vi "Control Panel Controller.vi"(8 "error in (no error)":errorcluster, 11 "Control Panel in":refnum<class "Control Panel.lvclass">) -> (0 "error out":errorcluster, 2 "Solenoid":bool, 3 "Control Panel out":refnum<class "Control Panel.lvclass">)   [LabVIEW 2019, in "Control Panel.lvlib" / "Control Panel.lvclass"]
uses:
  Control Panel.lvclass
  Controls/Control Panel State.ctl
panel:
  in  "Rotation":bool
  in  "Position":bool
  in  "Manual":dbl
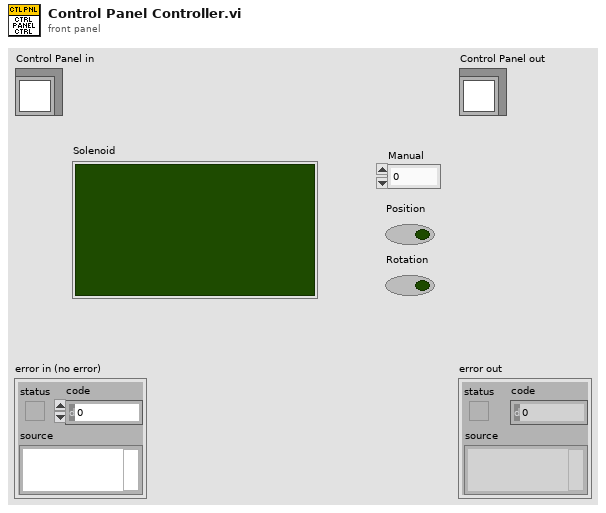
[diagram p1: front panel]
types:
  T1 = typedef "Control Panel State.ctl" = enum16{"Manual Control", "Position Control", "Rotation Control", "Retracted", "Deployed"}
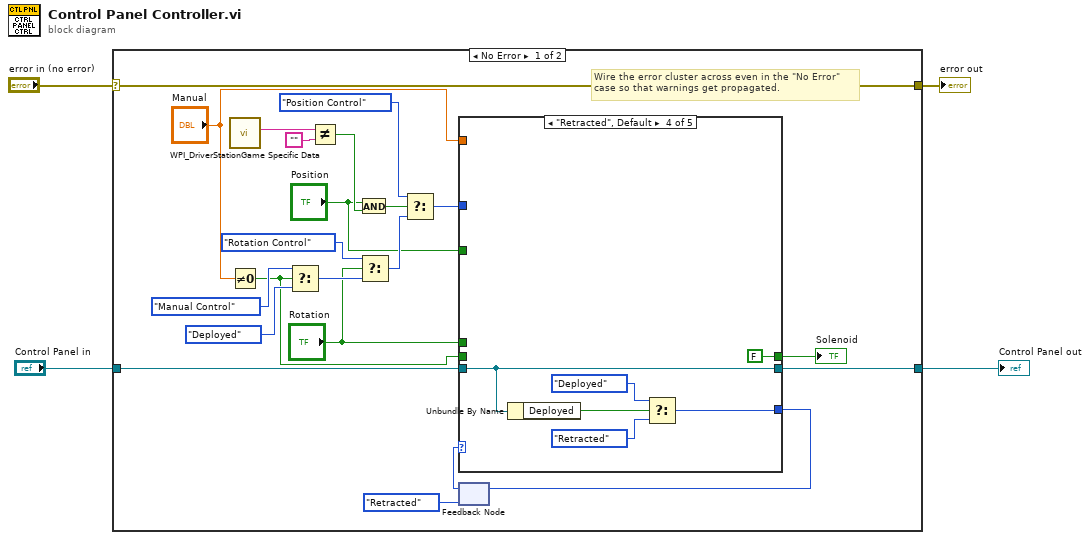
[diagram p0: block diagram]
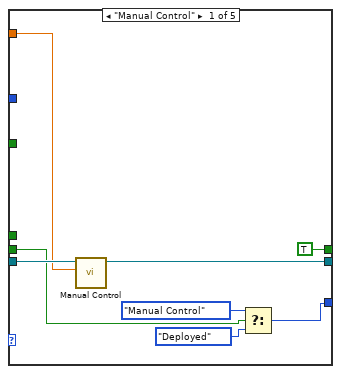
[diagram p2: hidden frame]
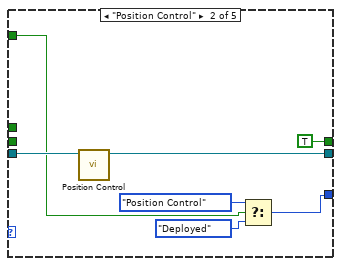
[diagram p3: hidden frame]
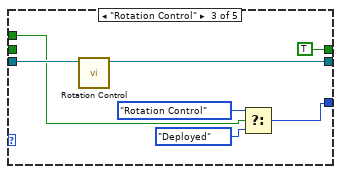
[diagram p4: hidden frame]
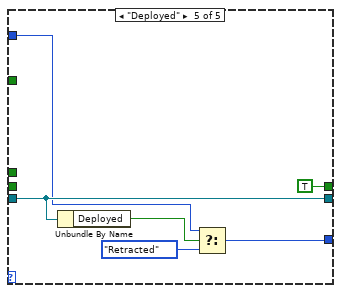
[diagram p5: hidden frame]
diagram:
  n1 = case shown="No Error" "error in (no error)" {
    selector: "error in (no error)" -> [w26 w62]
    tunnel: [w26 w62] -> w3
    tunnel: [w22 w61] -> w1
    tunnel: "Control Panel in" -> [w23 w61]
    frame No Error {
      # "Wire the error cluster across even in the \"No Error\"\ncase so that warnings get propagated."
      n2 = call <vilib>:"WPI_DriverStationGame Specific Data.vi"() -> ("Game Specific Data"=w13:string)  [unwired: 11 in]
      n3 = Not Equal To 0?(x="Manual") -> (x != 0?=w6:bool)
      n4 = Select(t=Control_Panel_State."Manual Control", s=w6, f=Control_Panel_State."Deployed") -> (s? t:f=w18:T1)
      n5 = Not Equal?(x=w13, y="") -> (x != y?=w11:bool)
      n6 = And(x="Position", y=w11) -> (x .and. y?=w5:bool)
      n7 = Select(t=Control_Panel_State."Rotation Control", s="Rotation", f=w18) -> (s? t:f=w19:T1)
      n8 = Select(t=Control_Panel_State."Position Control", s=w5, f=w19) -> (s? t:f=w10:T1)
      n9 = feedback #1(Control_Panel_State."Retracted") -> (w24:T1)
      n10 = case shown="\"Retracted\", Default" w24 {
        tunnel: w23 -> [w34 w41 w48 w51 w59]
        tunnel: [w27 w37 w42 w51 w59] -> w22
        tunnel: [w29 w38 w44 w54 w55] -> w20
        tunnel: [TRUE ("Deployed") TRUE ("Deployed") TRUE ("Deployed") FALSE ("Deployed") TRUE ("Deployed")] -> w21
        tunnel: w10 -> [_ _ _ _ w56]
        tunnel: "Rotation" -> [_ _ w47 _ _]
        tunnel: "Position" -> [_ w36 _ _ _]
        tunnel: "Manual" -> [w33 _ _ _ _]
        tunnel: w6 -> [w32 _ _ _ _]
        frame "Manual Control" {
          n11 = call-dynamic "Manual Control.vi"("Output"=w33, "Control Panel in"=w34) -> ("Control Panel out"=w27:refnum<class "Control Panel.lvclass">)  [unwired: 8 in, 1 out]
          n12 = Select(t=Control_Panel_State."Manual Control", s=w32, f=Control_Panel_State."Deployed") -> (s? t:f=w29:T1)
        }
        frame "Position Control" {
          n13 = call-dynamic "Position Control.vi"("Control Panel in"=w41) -> ("Control Panel out"=w37:refnum<class "Control Panel.lvclass">)  [unwired: 9 in, 1 out]
          n14 = Select(t=Control_Panel_State."Position Control", s=w36, f=Control_Panel_State."Deployed") -> (s? t:f=w38:T1)
        }
        frame "Rotation Control" {
          n15 = call-dynamic "Rotation Control.vi"("Control Panel in"=w48) -> ("Control Panel out"=w42:refnum<class "Control Panel.lvclass">)  [unwired: 9 in, 1 out]
          n16 = Select(t=Control_Panel_State."Rotation Control", s=w47, f=Control_Panel_State."Deployed") -> (s? t:f=w44:T1)
        }
        frame "Retracted", Default {
          n17 = Unbundle By Name(w51) -> ("Deployed"=w50:bool)
          n18 = Select(t=Control_Panel_State."Deployed", s=w50, f=Control_Panel_State."Retracted") -> (s? t:f=w54:T1)
        }
        frame "Deployed" {
          n19 = Unbundle By Name(w59) -> ("Deployed"=w58:bool)
          n20 = Select(t=w56, s=w58, f=Control_Panel_State."Retracted") -> (s? t:f=w55:T1)
        }
      }
      "Solenoid" <- w21
      n21 = feedback-in #1(w20) -> ()
    }
    frame Error {
    }
  }
  "error out" <- w3
  "Control Panel out" <- w1
